vi "Create Chans.vi"(4 "Minimum Value":T4, 5 "Sensor Type":T1, 6 "Maximum Value":T3, 7 "# of Chans":u8, 8 "error in":errorcluster, 9 "scaling information":variant, 10 "bridge information":variant, 11 "Item Ref in":T2 format="%.0x") -> (0 "error out":errorcluster, 3 "Item Ref out":T2 format="%.0x")   [LabVIEW 2010, in "PXIe-433x Custom Device.lvlib"]
uses:
  PXIe-433x Custom Device.lvlib
  Min Value.ctl
  Max Value.ctl
  <vilib>/NI VeriStand/Custom Device API/Custom Device Item Ref.ctl
  Sensor Type.ctl
  <vilib>/NI VeriStand/Custom Device API/Custom Device Channel.ctl
  <vilib>/NI VeriStand/Custom Device API/Custom Device Channel Type.ctl
  Force Scaling Information.ctl
  Pressure Scaling Information.ctl
  Torque Scaling Information.ctl
  Global.vi
  <vilib>/NI Veristand/Custom Device Tools/Custom Device Utility Library/NI VeriStand - Search for All Items by GUID.vi
  <vilib>/NI VeriStand/Custom Device API/Get Item Property (U16).vi
  <vilib>/NI VeriStand/Custom Device API/Set Item Property (U16).vi
  <vilib>/NI Veristand/Custom Device API/Custom Device API.lvlib
  <vilib>/NI Veristand/Custom Device Tools/Custom Device Utility Library/Custom Device Utility Library.lvlib
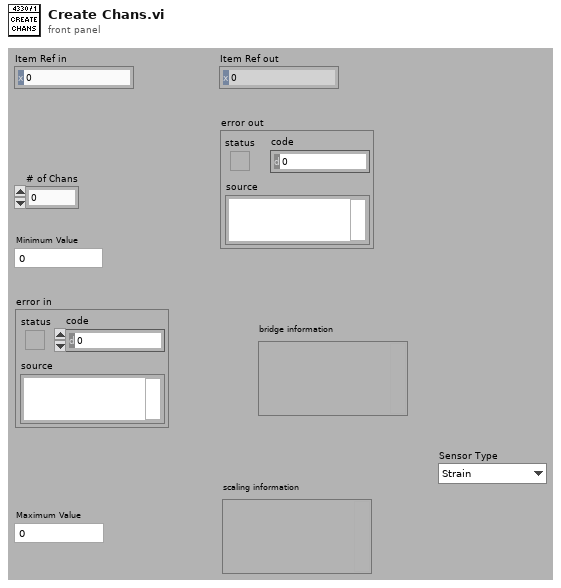
[diagram p1: front panel]
types:
  T1 = typedef "PXIe-433x Custom Device.lvlib/Sensor Type.ctl" = enum16{"Strain", "Force", "Pressure", "Torque"}
  T2 = typedef "Custom Device API.lvlib/Custom Device Item Ref.ctl" = u64
  T3 = typedef "PXIe-433x Custom Device.lvlib/Max Value.ctl" = dbl
  T4 = typedef "PXIe-433x Custom Device.lvlib/Min Value.ctl" = dbl
  T5 = typedef "Custom Device API.lvlib/Custom Device Channel.ctl" = cluster{"Type":T6, "Units":string, "Default Value":dbl, "Faultable":bool, "Scalable":bool}
  T6 = typedef "Custom Device API.lvlib/Custom Device Channel Type.ctl" = enum16{"Input", "Output"}
  T7 = typedef "PXIe-433x Custom Device.lvlib/Force Scaling Information.ctl" = cluster{"first electrical value":dbl, "second electrical value":dbl, "electrical units":i32, "first physical value":dbl, "second physical value":dbl, "physical units":i32}
  T8 = typedef "PXIe-433x Custom Device.lvlib/Pressure Scaling Information.ctl" = cluster{"first electrical value":dbl, "second electrical value":dbl, "electrical units":i32, "first physical value":dbl, "second physical value":dbl, "physical units":i32}
  T9 = typedef "PXIe-433x Custom Device.lvlib/Torque Scaling Information.ctl" = cluster{"first electrical value":dbl, "second electrical value":dbl, "electrical units":i32, "first physical value":dbl, "second physical value":dbl, "physical units":i32}
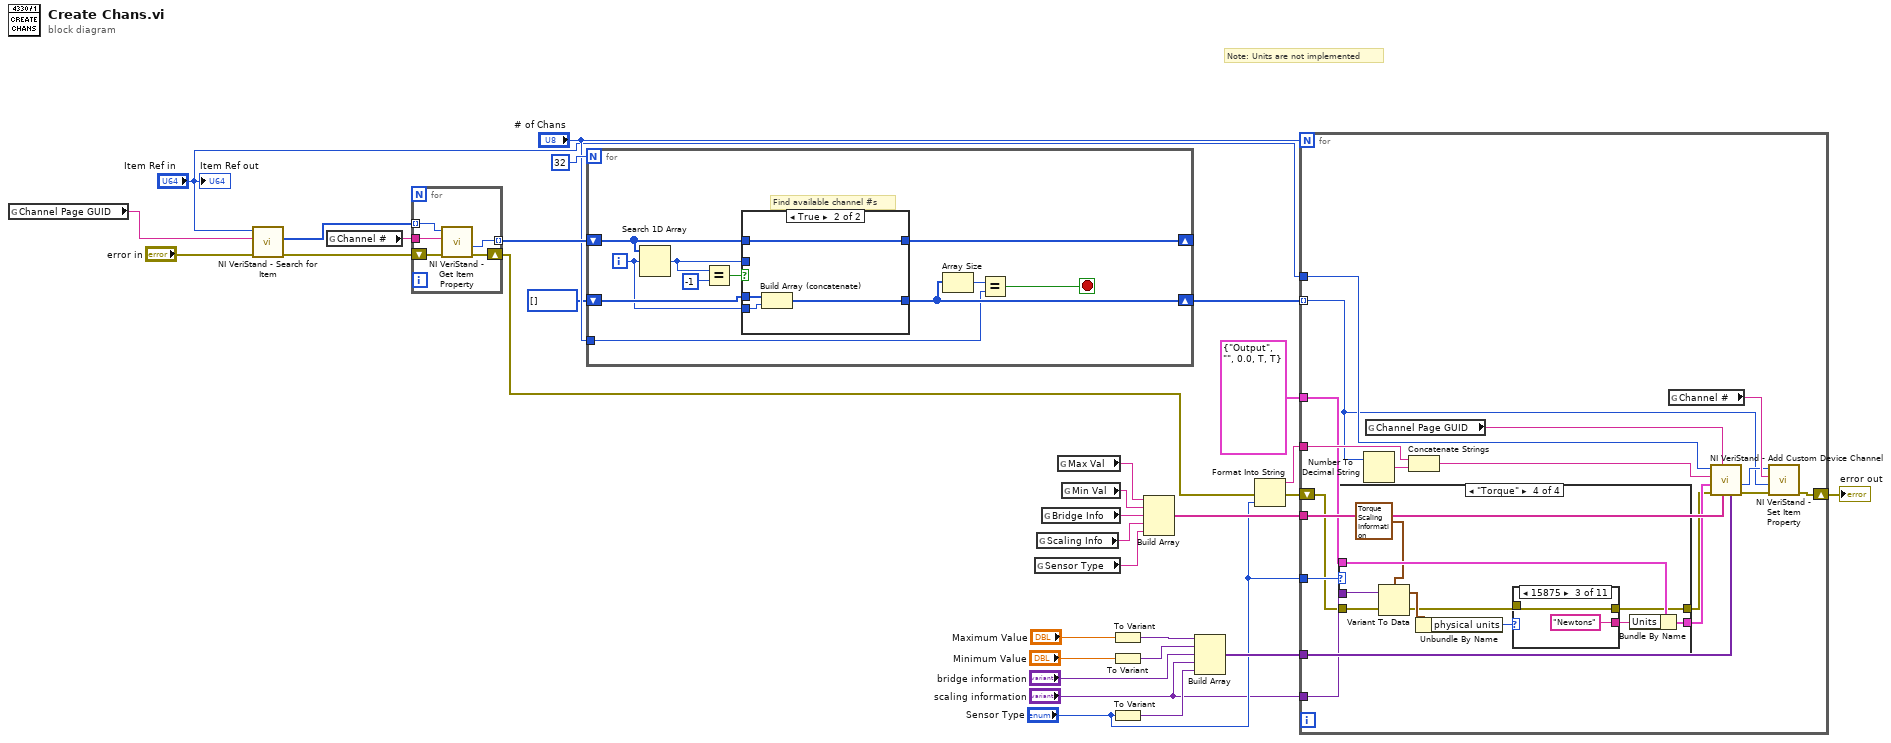
[diagram p0: block diagram]
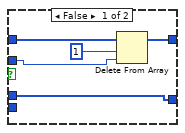
[diagram p2: hidden frame]
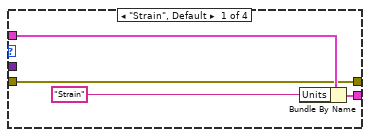
[diagram p3: hidden frame]
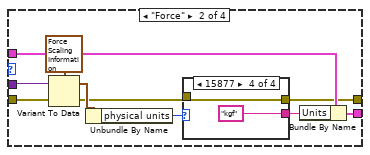
[diagram p4: hidden frame]
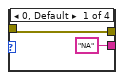
[diagram p5: hidden frame]
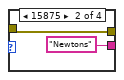
[diagram p6: hidden frame]
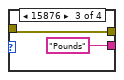
[diagram p7: hidden frame]
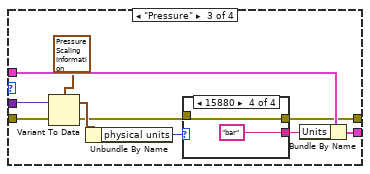
[diagram p8: hidden frame]
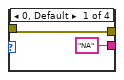
[diagram p9: hidden frame]
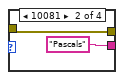
[diagram p10: hidden frame]
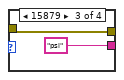
[diagram p11: hidden frame]
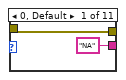
[diagram p12: hidden frame]
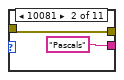
[diagram p13: hidden frame]
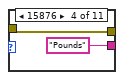
[diagram p14: hidden frame]
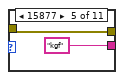
[diagram p15: hidden frame]
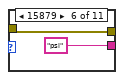
[diagram p16: hidden frame]
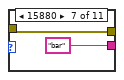
[diagram p17: hidden frame]
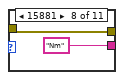
[diagram p18: hidden frame]
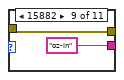
[diagram p19: hidden frame]
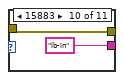
[diagram p20: hidden frame]
diagram:
  # "Note: Units are not implemented"
  n1 = global read "Global.vi" "Channel Page GUID"() -> (w3:string)
  n2 = call-poly <vilib>:"NI VeriStand - Search for Item.vi"("error in"="error in", "Item GUID"=w3, "Section Ref in"="Item Ref in") -> ("error out"=w6:errorcluster, "Item Refs"=w5:T2[])  [unwired: 5 in, 2 out]
  n3 = global read "Global.vi" "Channel #"() -> (w21:string)
  n4 = for {
    tunnel: w5 -> [w36] mode=indexing
    shift-right: [w33] -> w10
    shift-left: w6 -> [w35]
    tunnel: w21 -> [w34]
    tunnel: [w32] -> w20 mode=indexing
    n5 = call-poly <vilib>:"NI VeriStand - Get Item Property.vi"("error in (no error)"=w35, "Property Name"=w34, "Item Ref in"=w36) -> ("error out"=w33:errorcluster, "Value"=w32:u16)  [unwired: 5 in, 2 out]
  }
  n6 = for {
    N: 32 -> [_]
    shift-right: [w40] -> w19
    shift-left: i32[] [] -> [w45]
    shift-right: [w41] -> _
    shift-left: w20 -> [w43]
    tunnel: "# of Chans" -> [w38]
    i -> [w44]
    stop <- w37 stop-if-true
    # "Find available channel #s"
    n7 = Search 1D Array(1D array=w43, element=w44) -> (index of element=w42:i32)  [unwired: 1 in]
    n8 = Equal?(x=w42, y=-1) -> (x = y?=w46:bool)
    n9 = case shown="True" w46 {
      tunnel: w45 -> [w52 w56]
      tunnel: [w52 w55] -> w40
      tunnel: w44 -> [_ w54]
      tunnel: w43 -> [w51 w53]
      tunnel: w42 -> [w49 _]
      tunnel: [w48 w53] -> w41
      frame False {
        n10 = Delete From Array(array=w51, length=1, index=w49) -> (array with subset deleted=w48:u16[])  [unwired: 1 out]
      }
      frame True {
        n11 = Build Array (concatenate)(w56, w54) -> (w55:i32[])
      }
    }
    n12 = Array Size(array=w40) -> (size(s)=w39:i32)
    n13 = Equal?(x=w39, y=w38) -> (x = y?=w37:bool)
  }
  n14 = global read "Global.vi" "Sensor Type"() -> (w13:string)
  n15 = global read "Global.vi" "Scaling Info"() -> (w15:string)
  n16 = global read "Global.vi" "Bridge Info"() -> (w16:string)
  n17 = global read "Global.vi" "Max Val"() -> (w24:string)
  n18 = global read "Global.vi" "Min Val"() -> (w25:string)
  n19 = To Variant(anything="Maximum Value") -> (Variant=w28:variant)
  n20 = To Variant(anything="Minimum Value") -> (Variant=w29:variant)
  n21 = To Variant(anything="Sensor Type") -> (Variant=w12:variant)
  n22 = Build Array(w24, w25, w16, w15, w13) -> (w31:string[])
  n23 = Build Array(w28, w29, "bridge information", "scaling information", w12) -> (w30:variant[])
  n24 = Format Into String(error in=w10, "Sensor Type") -> (resulting string=w11:string, error out=w9:errorcluster)  [unwired: 2 in]
  n25 = for {
    N: "# of Chans" -> [_]
    shift-right: [w63] -> w23
    shift-left: w9 -> [w58]
    tunnel: T5 {"Type"=enum."Output", "Units"="", "Default Value"=0.0, "Faultable"=TRUE, "Scalable"=TRUE} ("Channel") -> [w61]
    tunnel: "Item Ref in" -> [w74]
    tunnel: w11 -> [w73]
    tunnel: w30 -> [w66]
    tunnel: w31 -> [w65]
    tunnel: w19 -> [w64] mode=indexing
    tunnel: "Sensor Type" -> [w62]
    tunnel: "scaling information" -> [w60]
    n26 = case shown="\"Torque\"" w62 {
      tunnel: w61 -> [w78 w88 w106 w124]
      tunnel: w60 -> [_ w86 w104 w122]
      tunnel: [w77 w87 w105 w123] -> w59
      tunnel: w58 -> [w75 w85 w103 w121]
      tunnel: [w75 w80 w98 w117] -> w57
      frame "Strain", Default {
        n27 = Bundle By Name(cluster=w78, "Units"="Strain") -> (w77:T5)
      }
      frame "Force" {
        n28 = Variant To Data(error in=w85, Variant=w86, type=T7 {"first electrical value"=0.0, "second electrical value"=2.0, "electrical units"=15897, "first physical value"=0.0, "second physical value"=100.0, "physical units"=15876} ("scaling information")) -> (error out=w82:errorcluster, data=w83:T7)
        n29 = Unbundle By Name(w83) -> ("physical units"=w81:i32)
        n30 = case shown="15877" w81 {
          tunnel: w82 -> [w90 w91 w93 w95]
          tunnel: [w90 w91 w93 w95] -> w80
          tunnel: ["NA" "Newtons" "Pounds" "kgf"] -> w79
          frame 0, Default {
          }
          frame 15875 {
          }
          frame 15876 {
          }
          frame 15877 {
          }
        }
        n31 = Bundle By Name(cluster=w88, "Units"=w79) -> (w87:T5)
      }
      frame "Pressure" {
        n32 = Variant To Data(error in=w103, Variant=w104, type=T8 {"first electrical value"=0.0, "second electrical value"=2.0, "electrical units"=15897, "first physical value"=0.0, "second physical value"=100.0, "physical units"=10081} ("scaling information")) -> (error out=w100:errorcluster, data=w101:T8)
        n33 = Unbundle By Name(w101) -> ("physical units"=w99:i32)
        n34 = case shown="15880" w99 {
          tunnel: w100 -> [w108 w109 w111 w113]
          tunnel: [w108 w109 w111 w113] -> w98
          tunnel: ["NA" "Pascals" "psi" "bar"] -> w97
          frame 0, Default {
          }
          frame 10081 {
          }
          frame 15879 {
          }
          frame 15880 {
          }
        }
        n35 = Bundle By Name(cluster=w106, "Units"=w97) -> (w105:T5)
      }
      frame "Torque" {
        n36 = Variant To Data(error in=w121, Variant=w122, type=T9 {"first electrical value"=0.0, "second electrical value"=2.0, "electrical units"=15897, "first physical value"=0.0, "second physical value"=100.0, "physical units"=15883} ("scaling information")) -> (error out=w119:errorcluster, data=w120:T9)
        n37 = Unbundle By Name(w120) -> ("physical units"=w118:i32)
        n38 = case shown="15875" w118 {
          tunnel: w119 -> [w126 w127 w129 w131 w133 w135 w137 w139 w141 w143 w145]
          tunnel: [w126 w127 w129 w131 w133 w135 w137 w139 w141 w143 w145] -> w117
          tunnel: ["NA" "Pascals" "Newtons" "Pounds" "kgf" "psi" "bar" "Nm" "oz-in" "lb-in" "lb-ft"] -> w116
          frame 0, Default {
          }
          frame 10081 {
          }
          frame 15875 {
          }
          frame 15876 {
          }
          frame 15877 {
          }
          frame 15879 {
          }
          frame 15880 {
          }
          frame 15881 {
          }
          frame 15882 {
          }
          frame 15883 {
          }
          frame 15884 {
          }
        }
        n39 = Bundle By Name(cluster=w124, "Units"=w116) -> (w123:T5)
      }
    }
    n40 = Number To Decimal String(number=w64) -> (decimal integer string=w72:string)  [unwired: 1 in]
    n41 = global read "Global.vi" "Channel Page GUID"() -> (w70:string)
    n42 = Concatenate Strings(w73, w72) -> (w71:string)
    n43 = global read "Global.vi" "Channel #"() -> (w68:string)
    n44 = call <vilib>:"NI VeriStand - Add Custom Device Channel.vi"("Property Values"=w66, "Property names"=w65, "GUID (Default Channel)"=w70, "error in (no error)"=w57, "Channel"=w59, "Channel Name"=w71, "Parent Ref in"=w74) -> ("error out"=w69:errorcluster, "Channel Ref"=w67:T2)  [unwired: 1 in, 2 out]
    n45 = call-poly <vilib>:"NI VeriStand - Set Item Property.vi"("error in (no error)"=w69, "Value"=w64, "Property Name"=w68, "Item Ref in"=w67) -> ("error out"=w63:errorcluster)  [unwired: 5 in, 2 out]
  }
  "error out" <- w23
  "Item Ref out" <- "Item Ref in"
